vi "Get Transfer UIs.vi"(8 "error in (no error)":errorcluster, 11 "Component UI in":refnum<class "UDP User Interfaces.lvclass">) -> (0 "error out":errorcluster, 1 "Tx Transfer UI":refnum<class "User Interface.lvclass">, 2 "Rx Transfer UI":refnum<class "User Interface.lvclass">, 3 "Component UI out":refnum<class "UDP User Interfaces.lvclass">)   [LabVIEW 2023, in "UDP.lvlib" / "UDP User Interfaces.lvclass"]
uses:
  UDP User Interfaces.lvclass
  Users/Public/Documents/National Instruments/NI VeriStand 2023/Custom Devices/Data Sharing Framework/Linux_x64/DSF Core.lvlibp/Classes/User Interface/User Interface.lvclass
  Transfer Tx/UDP Transfer Tx User Interface.lvclass
  C:/Users/Public/Documents/National Instruments/NI VeriStand 2023/Custom Devices/Data Sharing Framework/Linux_x64/DSF Core.lvlibp/Classes/User Interface/User Interface.lvclass
  Transfer Rx/UDP Transfer Rx User Interface.lvclass
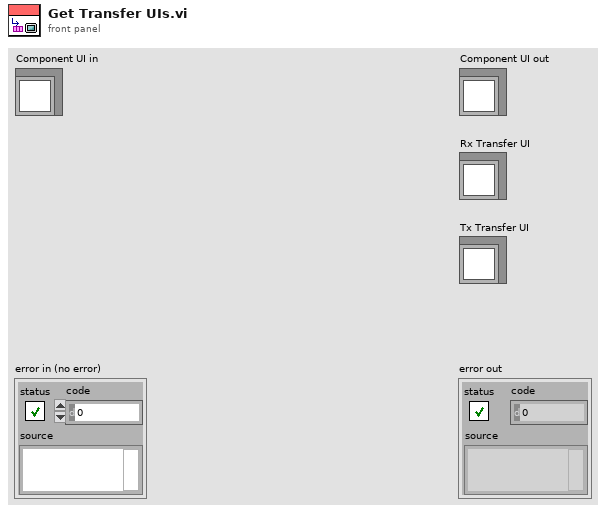
[diagram p1: front panel]
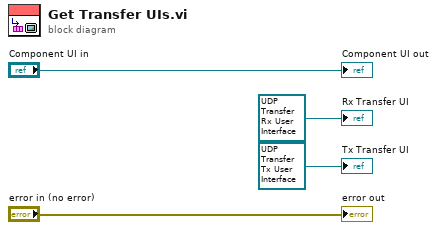
[diagram p0: block diagram]
diagram:
  "error out" <- "error in (no error)"
  "Component UI out" <- "Component UI in"
  "Rx Transfer UI" <- refnum<class "UDP Transfer Rx User Interface.lvclass"> refnum ("UDP Transceiver.lvlib:UDP Transfer Rx User Interface.lvclass")
  "Tx Transfer UI" <- refnum<class "UDP Transfer Tx User Interface.lvclass"> refnum ("UDP Transceiver.lvlib:UDP Transfer Tx User Interface.lvclass")
